vi "Apply special move.vi"(8 "error in (no error)":errorcluster, 10 "Position in":refnum<class "Position.lvclass">, 11 "DoublePush in":refnum<class "DoublePush.lvclass">) -> (0 "error out":errorcluster, 2 "Position out":refnum<class "Position.lvclass">, 3 "DoublePush out":refnum<class "DoublePush.lvclass">)   [LabVIEW 2015, in "Chesslib.lvlib" / "DoublePush.lvclass"]
uses:
  DoublePush.lvclass
  Position/Position.lvclass
  Move/Move.lvclass
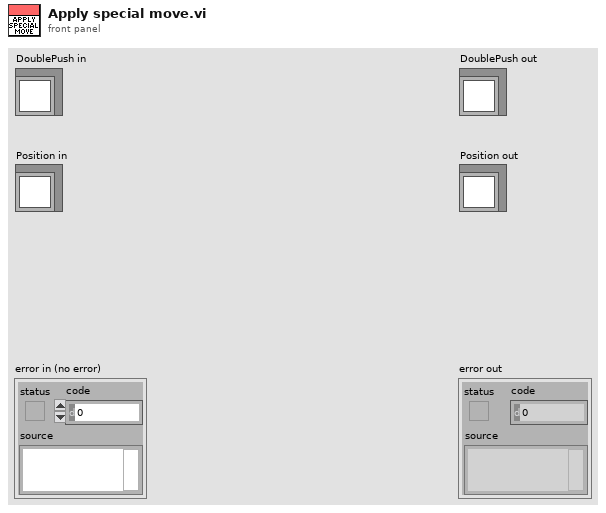
[diagram p1: front panel]
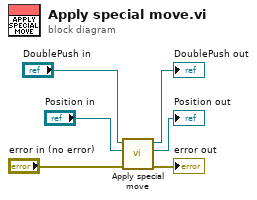
[diagram p0: block diagram]
diagram:
  n1 = call-parent "Apply special move.vi"("error in (no error)"="error in (no error)", "Position in"="Position in", "Move in"="DoublePush in") -> ("error out"=→"error out":errorcluster, "Position out"=→"Position out":refnum<class "Position.lvclass">, "Move out"=→"DoublePush out":refnum<class "DoublePush.lvclass">)  [unwired: 6 in]
